vi "setFPGAData.vi"(10 "TelemetryFPGAData":T1, 11 "Telemetry in":refnum<class "Telemetry.lvclass">) -> (3 "Telemetry out":refnum<class "Telemetry.lvclass">)   [LabVIEW 2016, in "Telemetry.lvclass"]
uses:
  Telemetry.lvclass
  Communicator/Topics/TelemetryFPGAData.ctl
  Types/Timestamp.ctl
  Telemetry.lvclass/Telemetry.ctl
  Types/M1M3SupportTypes.lvlib
  Communicator/M1M3Communicator.lvlib
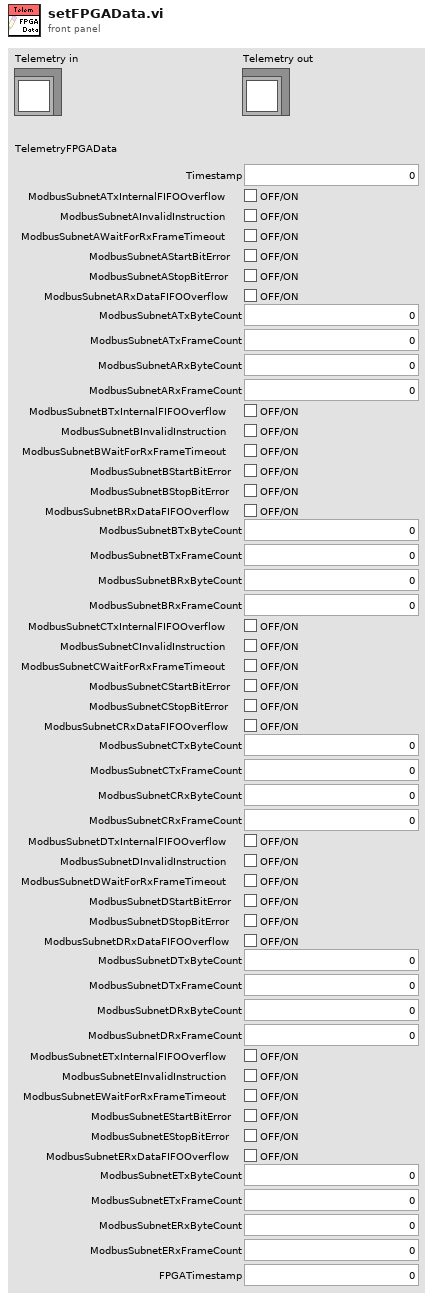
[diagram p1: front panel]
types:
  T1 = typedef "M1M3Communicator.lvlib/TelemetryFPGAData.ctl" = cluster{"Timestamp":T2, "ModbusSubnetATxInternalFIFOOverflow":bool, "ModbusSubnetAInvalidInstruction":bool, "ModbusSubnetAWaitForRxFrameTimeout":bool, "ModbusSubnetAStartBitError":bool, "ModbusSubnetAStopBitError":bool, "ModbusSubnetARxDataFIFOOverflow":bool, "ModbusSubnetATxByteCount":i32, "ModbusSubnetATxFrameCount":i32, "ModbusSubnetARxByteCount":i32, "ModbusSubnetARxFrameCount":i32, "ModbusSubnetBTxInternalFIFOOverflow":bool, "ModbusSubnetBInvalidInstruction":bool, "ModbusSubnetBWaitForRxFrameTimeout":bool, "ModbusSubnetBStartBitError":bool, "ModbusSubnetBStopBitError":bool, "ModbusSubnetBRxDataFIFOOverflow":bool, "ModbusSubnetBTxByteCount":i32, "ModbusSubnetBTxFrameCount":i32, "ModbusSubnetBRxByteCount":i32, "ModbusSubnetBRxFrameCount":i32, "ModbusSubnetCTxInternalFIFOOverflow":bool, "ModbusSubnetCInvalidInstruction":bool, "ModbusSubnetCWaitForRxFrameTimeout":bool, "ModbusSubnetCStartBitError":bool, "ModbusSubnetCStopBitError":bool, "ModbusSubnetCRxDataFIFOOverflow":bool, "ModbusSubnetCTxByteCount":i32, "ModbusSubnetCTxFrameCount":i32, "ModbusSubnetCRxByteCount":i32, "ModbusSubnetCRxFrameCount":i32, "ModbusSubnetDTxInternalFIFOOverflow":bool, "ModbusSubnetDInvalidInstruction":bool, "ModbusSubnetDWaitForRxFrameTimeout":bool, "ModbusSubnetDStartBitError":bool, "ModbusSubnetDStopBitError":bool, "ModbusSubnetDRxDataFIFOOverflow":bool, "ModbusSubnetDTxByteCount":i32, "ModbusSubnetDTxFrameCount":i32, "ModbusSubnetDRxByteCount":i32, "ModbusSubnetDRxFrameCount":i32, "ModbusSubnetETxInternalFIFOOverflow":bool, "ModbusSubnetEInvalidInstruction":bool, "ModbusSubnetEWaitForRxFrameTimeout":bool, "ModbusSubnetEStartBitError":bool, "ModbusSubnetEStopBitError":bool, "ModbusSubnetERxDataFIFOOverflow":bool, "ModbusSubnetETxByteCount":i32, "ModbusSubnetETxFrameCount":i32, "ModbusSubnetERxByteCount":i32, "ModbusSubnetERxFrameCount":i32, "FPGATimestamp":dbl}
  T2 = typedef "M1M3SupportTypes.lvlib/Timestamp.ctl" = dbl
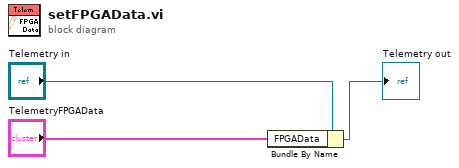
[diagram p0: block diagram]
diagram:
  n1 = Bundle By Name(cluster="Telemetry in", "FPGAData"="TelemetryFPGAData") -> (→"Telemetry out":refnum<class "Telemetry.lvclass">)
